vi "Write File.vi"(8 "error in":errorcluster, 10 "Data In":refnum<class "Data.lvclass">, 11 "File Obs in":refnum<class "cPAS File Obs.lvclass">) -> (0 "error out":errorcluster, 3 "File Obs out":refnum<class "cPAS File Obs.lvclass">)   [LabVIEW 2015, in "cPAS File Obs.lvclass"]
uses:
  cPAS File Obs.lvclass
  Reusable/Data/Data.lvclass
  Data/cPAS Data.lvclass
  Controls/MFC Address.ctl
  Controls/cPAS Data Enum.ctl
  Reusable/File IO/Class/File Observer.lvclass/File Observer.ctl
  Reusable/File IO/Class/Read File Ref.vi
  Data/Read Thum.vi
  Data/Read dcVolts.vi
  Reusable/PAS/File Observer/PAS File Obs.lvclass
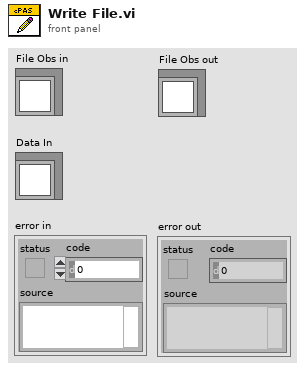
[diagram p1: front panel]
types:
  T1 = typedef "cPAS Data.lvclass/cPAS Data Enum.ctl" = u8
  T2 = typedef "MFC Address.ctl" = enum16{"CRDS Purge", "CRDS Thermodenuded", "CRDS Dry", "CRDS Med RH", "CRDS High RH", "PAS Ch 1", "PAS Ch 2", "PAS Ch3", "PAS Ch 4", "PAS Ch 5", "CLAP", "O3", "Pinlet"}
  T3 = enum16{"big-endian, network order", "native, host order", "little-endian"}
  T4 = cluster{"24V":sgl, "+15V":sgl, "- 15V":sgl, "12V":sgl, "Aux Volt":sgl}
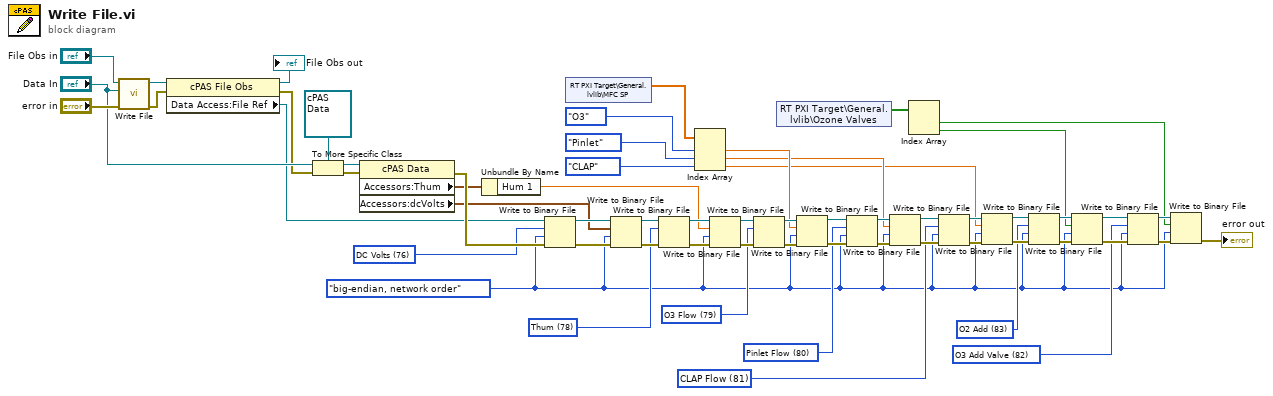
[diagram p0: block diagram]
diagram:
  w3 = T1 82 items=["DC Volts"=76, "T2"=77, "Thum"=78, "O3 Flow"=79, "Pinlet Flow"=80, "CLAP Flow"=81, "O3 Add Valve"=82, "O2 Add"=83] ("cPAS_Data_enum")
  w4 = T1 83 items=["DC Volts"=76, "T2"=77, "Thum"=78, "O3 Flow"=79, "Pinlet Flow"=80, "CLAP Flow"=81, "O3 Add Valve"=82, "O2 Add"=83] ("cPAS_Data_enum")
  w16 = T1 81 items=["DC Volts"=76, "T2"=77, "Thum"=78, "O3 Flow"=79, "Pinlet Flow"=80, "CLAP Flow"=81, "O3 Add Valve"=82, "O2 Add"=83] ("cPAS_Data_enum")
  w23 = T1 80 items=["DC Volts"=76, "T2"=77, "Thum"=78, "O3 Flow"=79, "Pinlet Flow"=80, "CLAP Flow"=81, "O3 Add Valve"=82, "O2 Add"=83] ("cPAS_Data_enum")
  w28 = T1 79 items=["DC Volts"=76, "T2"=77, "Thum"=78, "O3 Flow"=79, "Pinlet Flow"=80, "CLAP Flow"=81, "O3 Add Valve"=82, "O2 Add"=83] ("cPAS_Data_enum")
  w30 = T1 78 items=["DC Volts"=76, "T2"=77, "Thum"=78] ("cPAS_Data_enum")
  w31 = T1 76 items=["DC Volts"=76, "T2"=77, "Thum"=78] ("cPAS_Data_enum")
  w2 = T3."big-endian, network order" ("byte order (0:big-endian, network order)")
  n1 = call-parent "Write File.vi"("error in"="error in", "Data In"="Data In", "File Obs in"="File Obs in") -> ("error out"=w44:errorcluster, "File Obs out"=w45:refnum<class "cPAS File Obs.lvclass">)  [unwired: 7 in]
  n2 = property class="cPAS File Obs"(reference=w45, error in=w44) -> (reference out=→"File Obs out":refnum<class "cPAS File Obs.lvclass">, error out=w43:errorcluster, "Data Access:File Ref"=w40:refnum<file>)
  n3 = To More Specific Class(target class=refnum<class "cPAS Data.lvclass"> refnum ("cPAS Data"), reference="Data In", error in=w43) -> (specific class reference=w46:refnum<class "cPAS Data.lvclass">, error out=w41:errorcluster)
  n4 = property class="cPAS Data"(reference=w46, error in=w41) -> (error out=w58:errorcluster, "Accessors:Thum"=w50:cluster{"Hum 1":sgl, "Hum 2":sgl}, "Accessors:dcVolts"=w51:T4)  [unwired: 1 out]
  n5 = Unbundle By Name(w50) -> ("Hum 1"=w49:sgl)
  n6 = Write to Binary File(file (use dialog)=w40, data=w31, error in=w58, 9:w2) -> (refnum out=w57:refnum<file>, error out=w56:errorcluster)  [unwired: 2 in, 1 out]
  n7 = shared-variable "RT PXI Target\\General.lvlib\\MFC SP"() -> (w35:sgl[])  [unwired: 1 in, 1 out]
  n8 = Write to Binary File(file (use dialog)=w57, data=w51, error in=w56, 9:w2) -> (refnum out=w55:refnum<file>, error out=w54:errorcluster)  [unwired: 2 in, 1 out]
  n9 = Write to Binary File(file (use dialog)=w55, data=w30, error in=w54) -> (refnum out=w53:refnum<file>, error out=w52:errorcluster)  [unwired: 3 in, 1 out]
  n10 = Index Array(array=w35, index #1=MFC_Address."O3" ("Controllers"), index #2=MFC_Address."Pinlet" ("Controllers"), index #3=MFC_Address."CLAP" ("Controllers")) -> (element #1=w29:sgl, element #2=w22:sgl, element #3=w17:sgl)
  n11 = Write to Binary File(file (use dialog)=w53, data=w49, error in=w52, 9:w2) -> (refnum out=w39:refnum<file>, error out=w38:errorcluster)  [unwired: 2 in, 1 out]
  n12 = Write to Binary File(file (use dialog)=w39, data=w28, error in=w38) -> (refnum out=w37:refnum<file>, error out=w36:errorcluster)  [unwired: 3 in, 1 out]
  n13 = shared-variable "RT PXI Target\\General.lvlib\\Ozone Valves"() -> (w15:bool[])  [unwired: 1 in, 1 out]
  n14 = Write to Binary File(file (use dialog)=w37, data=w29, error in=w36, 9:w2) -> (refnum out=w24:refnum<file>, error out=w25:errorcluster)  [unwired: 2 in, 1 out]
  n15 = Write to Binary File(file (use dialog)=w24, data=w23, error in=w25, 9:w2) -> (refnum out=w26:refnum<file>, error out=w27:errorcluster)  [unwired: 2 in, 1 out]
  n16 = Write to Binary File(file (use dialog)=w26, data=w22, error in=w27, 9:w2) -> (refnum out=w19:refnum<file>, error out=w20:errorcluster)  [unwired: 2 in, 1 out]
  n17 = Index Array(array=w15) -> (element #1=w6:bool, element #2=w5:bool)  [unwired: 2 in]
  n18 = Write to Binary File(file (use dialog)=w19, data=w16, error in=w20, 9:w2) -> (refnum out=w21:refnum<file>, error out=w18:errorcluster)  [unwired: 2 in, 1 out]
  n19 = Write to Binary File(file (use dialog)=w21, data=w17, error in=w18, 9:w2) -> (refnum out=w11:refnum<file>, error out=w12:errorcluster)  [unwired: 2 in, 1 out]
  n20 = Write to Binary File(file (use dialog)=w11, data=w4, error in=w12, 9:w2) -> (refnum out=w13:refnum<file>, error out=w14:errorcluster)  [unwired: 2 in, 1 out]
  n21 = Write to Binary File(file (use dialog)=w13, data=w5, error in=w14, 9:w2) -> (refnum out=w7:refnum<file>, error out=w8:errorcluster)  [unwired: 2 in, 1 out]
  n22 = Write to Binary File(file (use dialog)=w7, data=w3, error in=w8, 9:w2) -> (refnum out=w10:refnum<file>, error out=w9:errorcluster)  [unwired: 2 in, 1 out]
  n23 = Write to Binary File(file (use dialog)=w10, data=w6, error in=w9, 9:w2) -> (error out=→"error out":errorcluster)  [unwired: 2 in, 2 out]
